vi "TCP Msg Write.vi"(7 "RT":bool, 8 "error in":errorcluster, 9 "timeout ms (10000)":i32=10000, 10 "Packet Info In":T1={"Packet Signature"="", "Sequence Number"=0, "Command"=enum."xml Set LC Input Logic", "Data Message Size"=0, "Data Message Size"="", "Data Message"="", "Error Message Size"=0, "Error Message Size"="", "Error Message"="", "Checksum"=0, "Error Message"={"status"=FALSE, "code"=0, "source"=""}, "Command ID"=""}, 11 "connection ID In":refnum<k5>) -> (0 "error out":errorcluster, 2 "Packet Info In Out":T1={"Packet Signature"="", "Sequence Number"=0, "Command"=enum."Get Info", "Data Message Size"=0, "Data Message Size"="", "Data Message"="", "Error Message Size"=0, "Error Message Size"="", "Error Message"="", "Checksum"=0, "Error Message"={"status"=FALSE, "code"=0, "source"=""}, "Command ID"=""}, 3 "connection ID out":refnum<k5>)   [LabVIEW 2018]
doc: "Writes a package of data to a remote computer via TCP/IP. The VI appends an ID number to each packet. This ID number is used by the Comm TCP Read VI to parse the packet using the meta data. This technique allows appending variable name and type to each packet for ease of use while minimizing the transmission overhead.\n\nThe data must be passed in as a String. The user is responsible for casting or flattening the desired data into a String before passing it to this VI. \n\n* Use the same method for converting to/from String on both the Read and Write functions. For example, if you use the 'Cast' primitive to convert the data into a String, make sure that the 'Cast' primitive is used on the receiving side to convert the data from String to its original form."
uses:
  Type Defs/TCP Packet Info.ctl
  Type Defs/RT Command.ctl
  Type Defs/TCP Packet Parsing State Machine.ctl
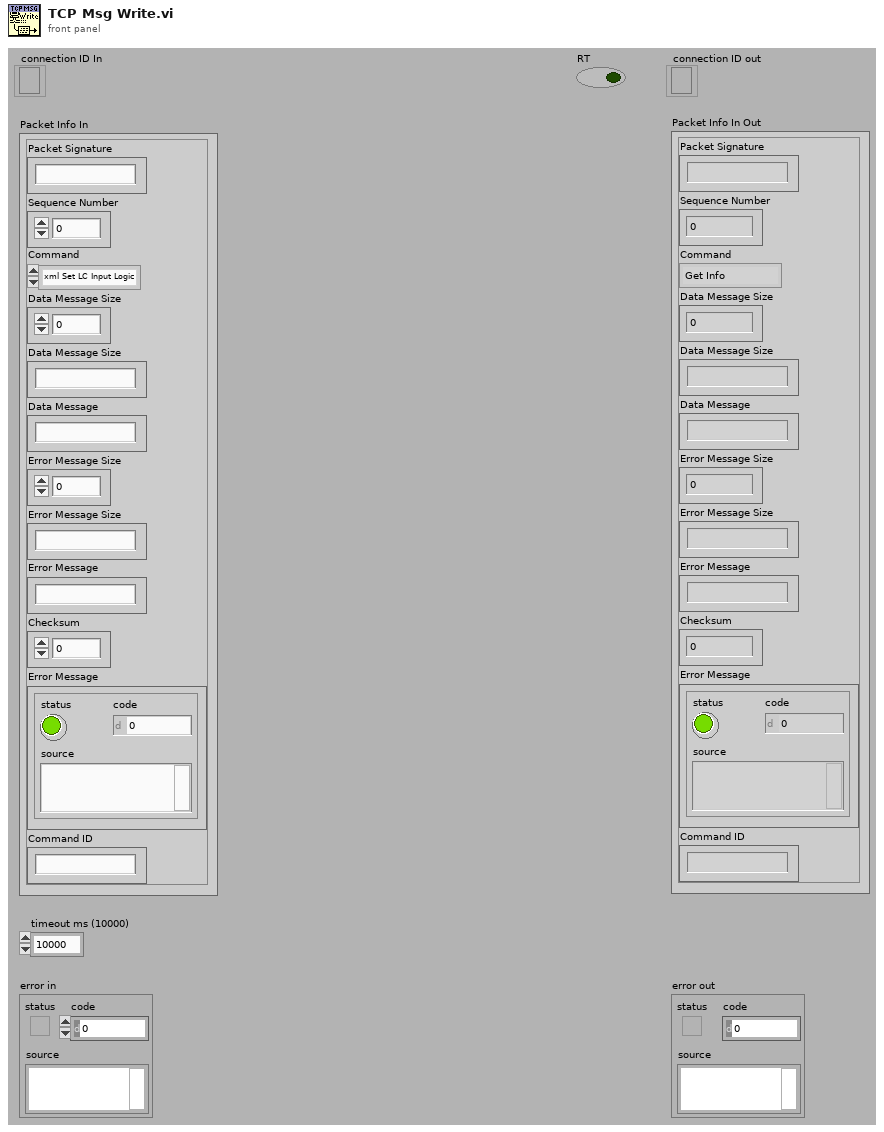
[diagram p1: front panel]
types:
  T1 = typedef "TCP Packet Info.ctl" = cluster{"Packet Signature":string, "Sequence Number":i32, "Command":T2, "Data Message Size":u32, "Data Message Size":string, "Data Message":string, "Error Message Size":u32, "Error Message Size":string, "Error Message":string, "Checksum":u32, "Error Message":errorcluster, "Command ID":string}
  T2 = typedef "RT Command.ctl" = enum16{"xml Start Run", "xml Start Actual Run", "xml Stop Run", "xml Runtime Update", "xml Get Status", "xml Get Table", "xml Set Table", "xml Get Configuration", "xml System Status", "xml Set LC Input Logic", "xml Get Data", "xml Get Info", "Start", "StartActualRun", "Stop", "Runtime Update", "Get Data", "Get Info", "Get Status", "Get Param", "Get Config", "Get Table", "Read ADC", "Set Oscillator", "Update Config", "Update Table", "Set All Pol", "Set Pol and DC", "Set Max Mass", "Toggle RP", "Toggle EL", "Set PIC", "Initialize Turbo", "Send Turbo Comm", "Close Turbo", "P1", "P2", "P3", "Send Serial", "Set LC Out", "Get LC In", "Read VAC", "Test Table", "Toggle Power", "Get Startup", "Set Startup", "Get ADC Table", "Set ADC Table", "Get Brief Status", "Get Detail Status", "Auxiliary Update", "Set CC Logics", "Set CC Input Logics", "Ignore Error", "invalid"}
  T3 = typedef "TCP Packet Parsing State Machine.ctl" = enum16{"Packet Signature", "Sequence Number", "Command ID", "Data Message Size", "Data Message", "Error Message Size", "Error Message", "Checksum", "Invalid Packet Structure"}
  T4 = enum16{"big-endian, network order", "native, host order", "little-endian"}
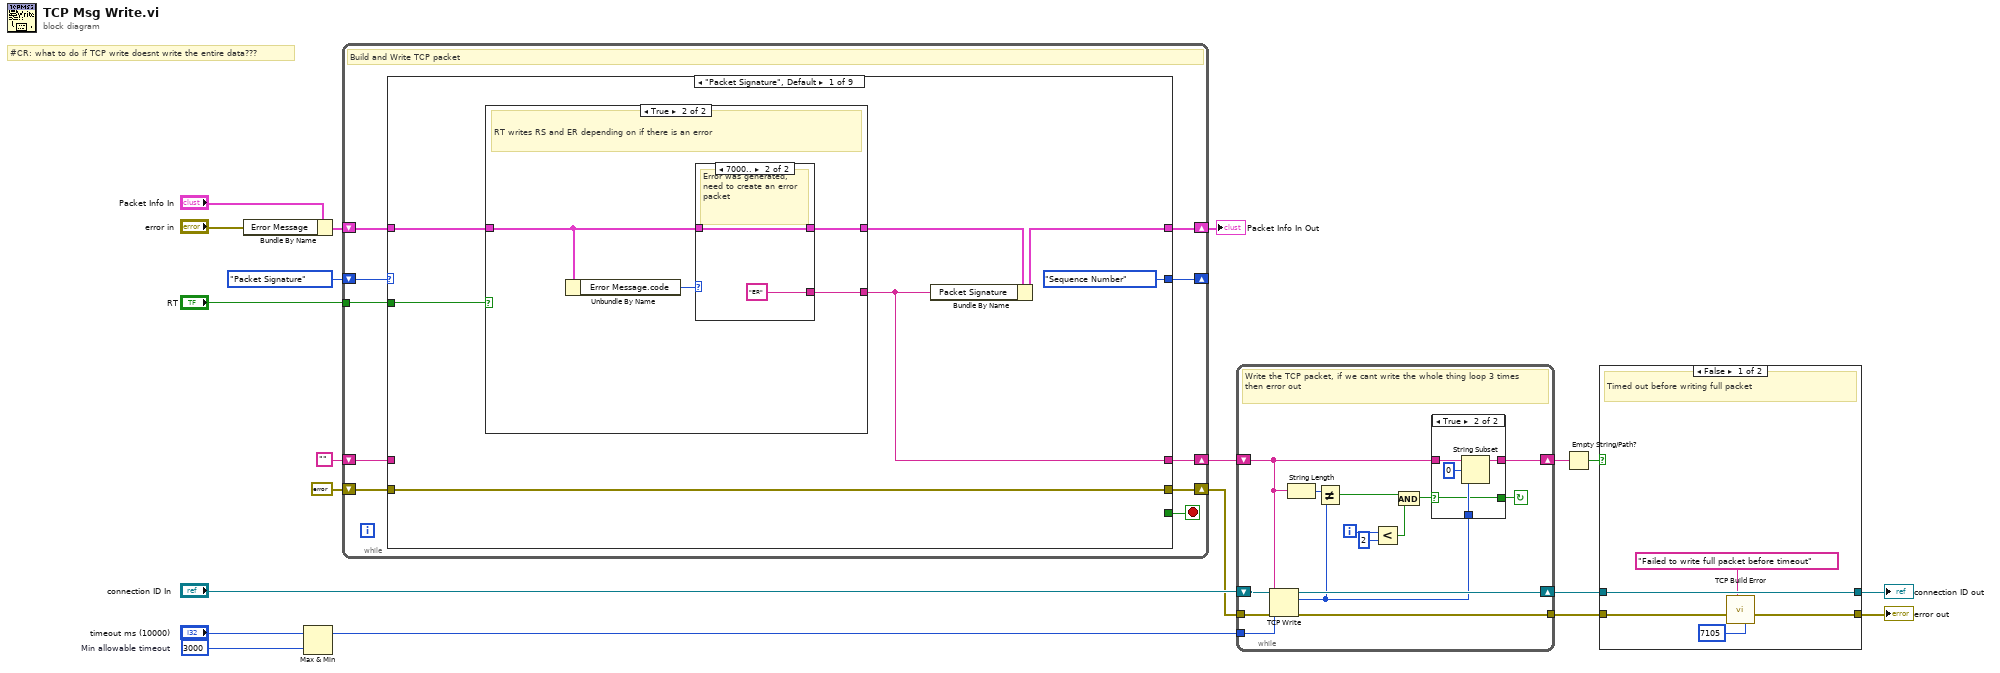
[diagram p0: block diagram]
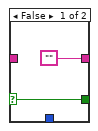
[diagram p3: hidden frame]
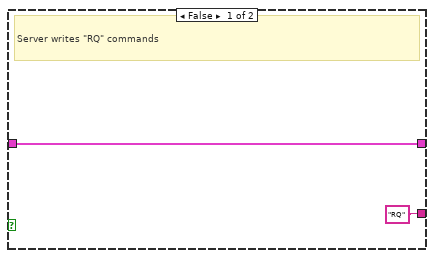
[diagram p4: hidden frame]
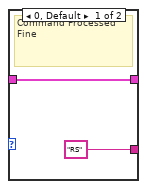
[diagram p5: hidden frame]
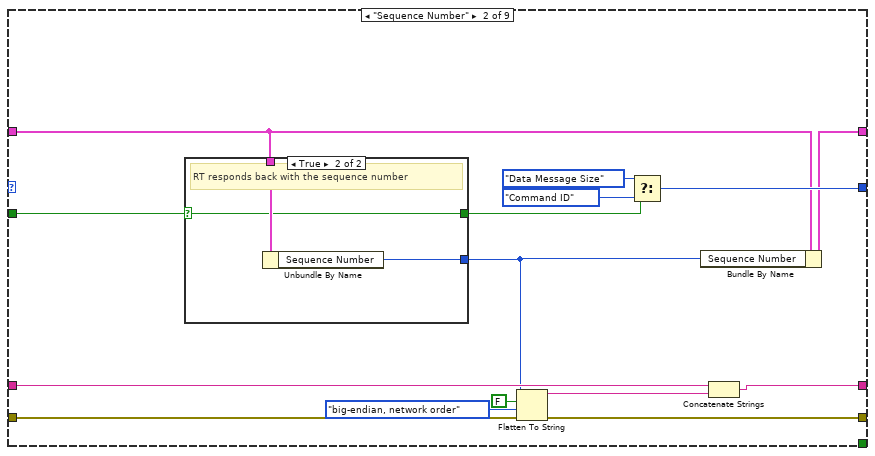
[diagram p6: hidden frame]
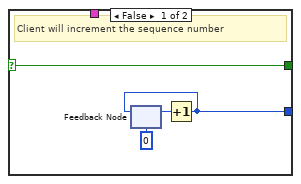
[diagram p7: hidden frame]
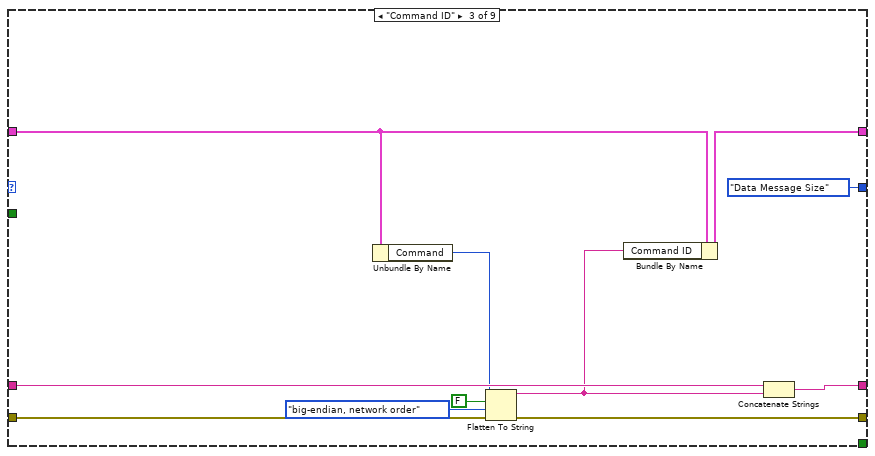
[diagram p8: hidden frame]
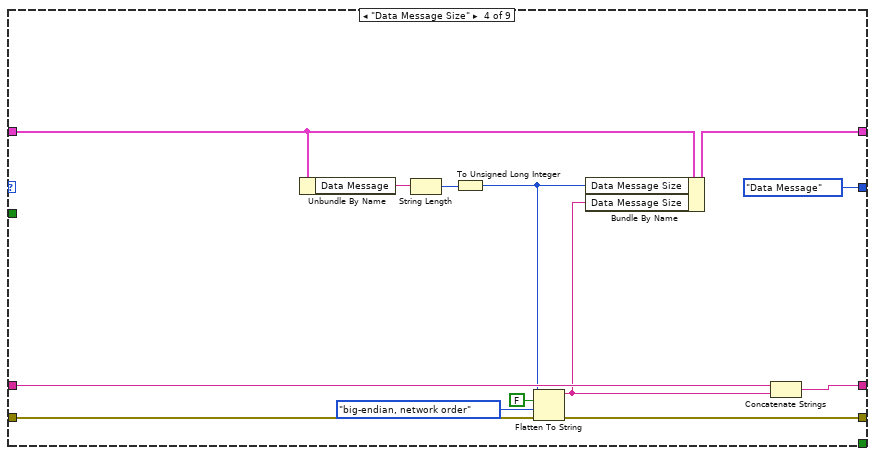
[diagram p9: hidden frame]
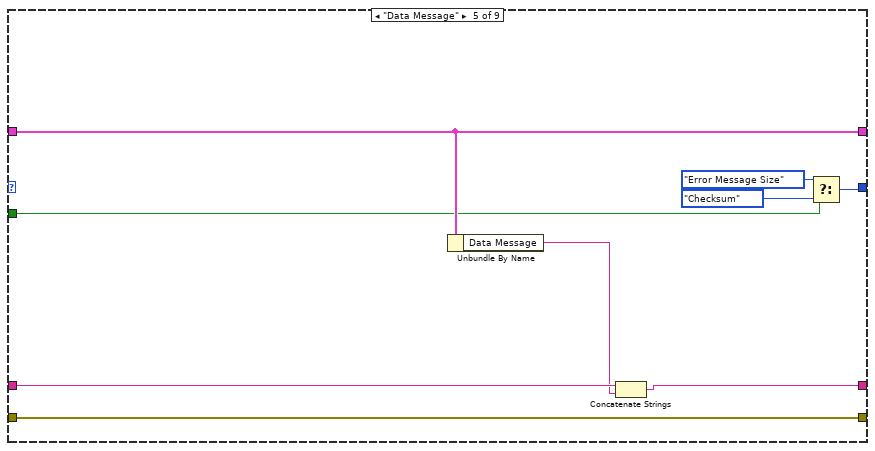
[diagram p10: hidden frame]
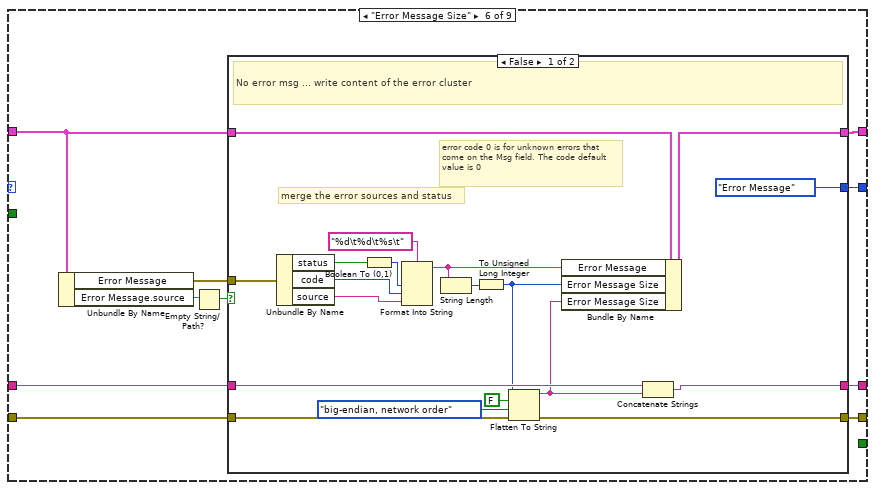
[diagram p11: hidden frame]
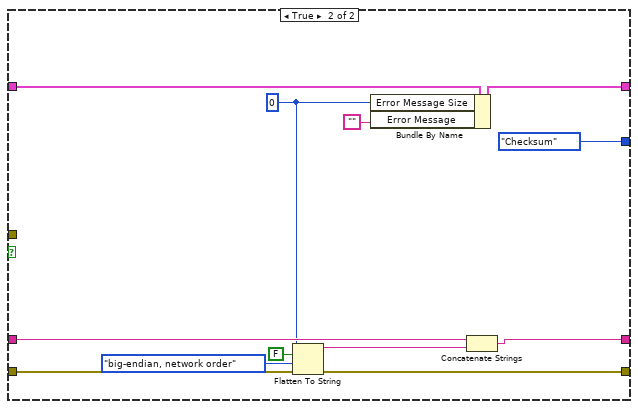
[diagram p12: hidden frame]
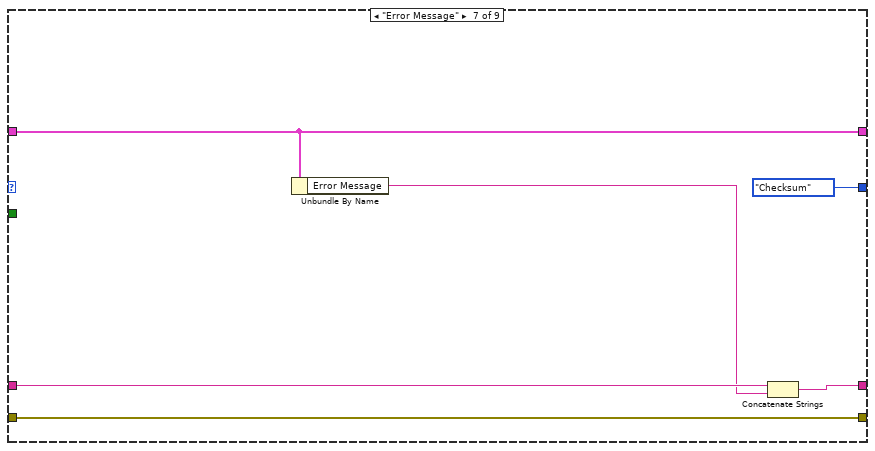
[diagram p13: hidden frame]
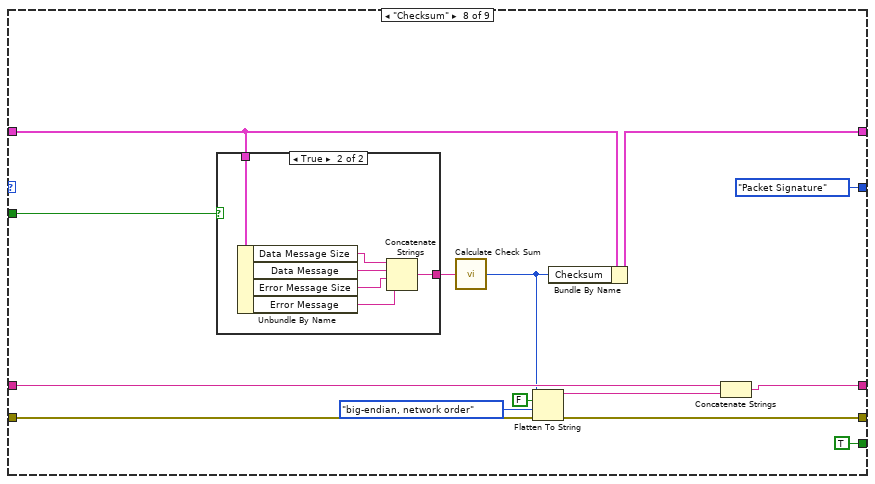
[diagram p14: hidden frame]
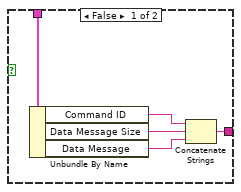
[diagram p15: hidden frame]
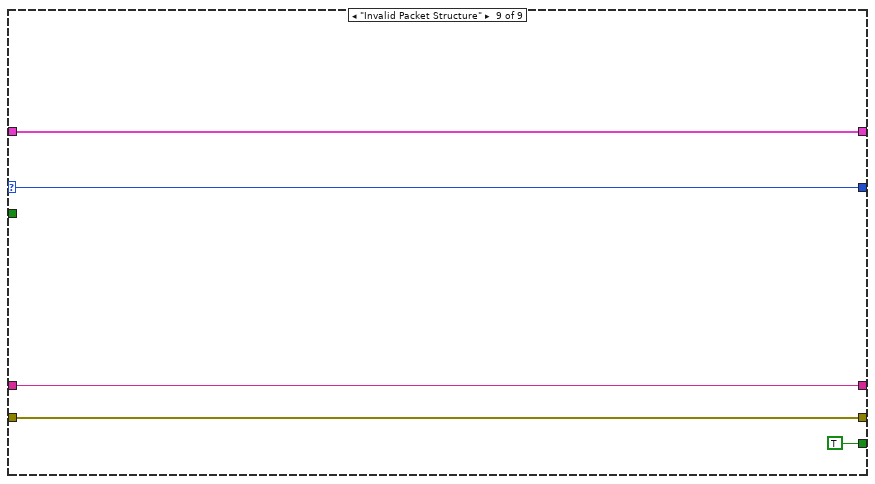
[diagram p16: hidden frame]
diagram:
  w16 = 3000  # Min allowable timeout
  # "#CR: what to do if TCP write doesnt write the entire data???"
  n1 = Bundle By Name(cluster="Packet Info In", "Error Message"="error in") -> (w15:T1)
  n2 = Max & Min(x="timeout ms (10000)", y=w16) -> (max(x,y)=w4:i32)  [unwired: 1 out]
  n3 = while {
    shift-right: [w29] -> w11
    shift-left: w15 -> [w30]
    tunnel: "RT" -> [w28]
    shift-right: [w27] -> _
    shift-left: TCP_Packet_Parsing_State_Machine."Packet Signature" ("Packet Structure") -> [w25]
    shift-right: [w23] -> w3
    shift-left: "" ("Message Packet") -> [w24]
    shift-right: [w21] -> w5
    shift-left: errorcluster {"status"=FALSE, "code"=0, "source"=""} ("error out") -> [w22]
    stop <- w26 stop-if-true
    # "Build and Write TCP packet"
    n4 = case shown="\"Packet Signature\", Default" w25 {
      selector: w25 -> [_ _ _ _ _ _ _ _ w177]
      tunnel: w30 -> [w35 w58 w80 w92 w102 w107 w149 w162 w179]
      tunnel: [w32 w49 w71 w83 w102 w108 w149 w163 w179] -> w29
      tunnel: w28 -> [w37 w59 _ _ w100 _ _ w159 _]
      tunnel: [TCP_Packet_Parsing_State_Machine."Sequence Number" ("Packet Structure") w61 TCP_Packet_Parsing_State_Machine."Data Message Size" ("Packet Structure") TCP_Packet_Parsing_State_Machine."Data Message" ("Packet Structure") w101 w111 TCP_Packet_Parsing_State_Machine."Checksum" ("Packet Structure") TCP_Packet_Parsing_State_Machine."Packet Signature" ("Packet Structure") w177] -> w27
      tunnel: [_ _ _ _ _ _ _ TRUE TRUE] -> w26
      tunnel: w24 -> [_ w56 w78 w88 w97 w106 w147 w157 w176]
      tunnel: [w31 w55 w77 w89 w96 w105 w146 w156 w176] -> w23
      tunnel: w22 -> [w33 w54 w74 w84 w94 w103 w144 w151 w175]
      tunnel: [w33 w51 w73 w85 w94 w104 w144 w153 w175] -> w21
      frame "Packet Signature", Default {
        # "Packet Header"
        n5 = case shown="True" w37 {
          tunnel: w35 -> [w39 w43]
          tunnel: [w39 w42] -> w36
          tunnel: ["RQ" ("data in") w41] -> w31
          frame False {
            # "Server writes \"RQ\" commands"
          }
          frame True {
            # "RT writes RS and ER depending on if there is an error"
            n6 = Unbundle By Name(w43) -> ("Error Message.code"=w40:i32)
            n7 = case shown="7000.." w40 {
              tunnel: w43 -> [w45 w47]
              tunnel: [w45 w47] -> w42
              tunnel: ["RS" ("data in") "ER" ("data in")] -> w41
              frame 0, Default {
                # "Command Processed Fine"
              }
              frame 7000.. {
                # "Error was generated, need to create an error packet"
              }
            }
          }
        }
        n8 = Bundle By Name(cluster=w36, "Packet Signature"=w31) -> (w32:T1)
      }
      frame "Sequence Number" {
        n9 = case shown="True" w59 {
          selector: w59 -> [w63 w67]
          tunnel: w58 -> [_ w69]
          tunnel: [w64 w68] -> w48
          tunnel: [w63 w67] -> w57
          frame False {
            # "Client will increment the sequence number"
            n10 = feedback #1(0 ("Sequence Number")) -> (w65:i32)
            n11 = Increment(x=w65) -> (x+1=w64:i32)
            n12 = feedback-in #1(w64) -> ()
          }
          frame True {
            # "RT responds back with the sequence number"
            n13 = Unbundle By Name(w69) -> ("Sequence Number"=w68:i32)
          }
        }
        n14 = Flatten To String(anything=w48, prepend array or string size? (T)=FALSE, byte order (0:big-endian, network order)=T4."big-endian, network order", error in (no error)=w54) -> (data string=w52:string, error out=w51:errorcluster)  [unwired: 1 out]
        n15 = Select(t=TCP_Packet_Parsing_State_Machine."Data Message Size" ("Packet Structure"), s=w57, f=TCP_Packet_Parsing_State_Machine."Command ID") -> (s? t:f=w61:T3)
        n16 = Bundle By Name(cluster=w58, "Sequence Number"=w48) -> (w49:T1)
        n17 = Concatenate Strings(w56, w52) -> (w55:string)
      }
      frame "Command ID" {
        n18 = Unbundle By Name(w80) -> ("Command"=w72:T2)
        n19 = Flatten To String(anything=w72, prepend array or string size? (T)=FALSE, byte order (0:big-endian, network order)=T4."big-endian, network order", error in (no error)=w74) -> (data string=w70:string, error out=w73:errorcluster)  [unwired: 1 out]
        n20 = Bundle By Name(cluster=w80, "Command ID"=w70) -> (w71:T1)
        n21 = Concatenate Strings(w78, w70) -> (w77:string)
      }
      frame "Data Message Size" {
        n22 = Unbundle By Name(w92) -> ("Data Message"=w91:string)
        n23 = String Length(string=w91) -> (length=w90:i32)
        n24 = To Unsigned Long Integer(number=w90) -> (unsigned 32bit integer=w82:u32)
        n25 = Flatten To String(anything=w82, prepend array or string size? (T)=FALSE ("data includes array or string size? (T)"), byte order (0:big-endian, network order)=T4."big-endian, network order", error in (no error)=w84) -> (data string=w81:string, error out=w85:errorcluster)  [unwired: 1 out]
        n26 = Bundle By Name(cluster=w92, "Data Message Size"=w82, "Data Message Size"=w81) -> (w83:T1)
        n27 = Concatenate Strings(w88, w81) -> (w89:string)
      }
      frame "Data Message" {
        n28 = Unbundle By Name(w102) -> ("Data Message"=w95:string)
        n29 = Concatenate Strings(w97, w95) -> (w96:string)
        n30 = Select(t=TCP_Packet_Parsing_State_Machine."Error Message Size" ("f"), s=w100, f=TCP_Packet_Parsing_State_Machine."Checksum" ("Packet Structure")) -> (s? t:f=w101:T3)
      }
      frame "Error Message Size" {
        n31 = Unbundle By Name(w107) -> ("Error Message"=w110:errorcluster, "Error Message.source"=w109:string)
        n32 = Empty String/Path?(string/path=w109) -> (empty?=w112:bool)
        n33 = case shown="False" w112 {
          tunnel: [TCP_Packet_Parsing_State_Machine."Error Message" ("Packet Structure") TCP_Packet_Parsing_State_Machine."Checksum" ("Packet Structure")] -> w111
          tunnel: w110 -> [w130 _]
          tunnel: [w124 w135] -> w108
          tunnel: w107 -> [w125 w142]
          tunnel: w106 -> [w120 w137]
          tunnel: [w119 w136] -> w105
          tunnel: [w117 w138] -> w104
          tunnel: w103 -> [w116 w139]
          frame False {
            # "error code 0 is for unknown errors that \ncome on the Msg field. The code default \nvalue is 0"
            # "merge the error sources and status"
            # "No error msg ... write content of the error cluster"
            n34 = Unbundle By Name(w130) -> ("status"=w121:bool, "code"=w127:i32, "source"=w126:string)
            n35 = Boolean To (0,1)(Boolean=w121) -> (0, 1=w128:i16)
            n36 = Format Into String(format string="%d\t%d\t%s\t", w128, w127, w126) -> (resulting string=w123:string)  [unwired: 2 in, 1 out]
            n37 = String Length(string=w123) -> (length=w122:i32)
            n38 = To Unsigned Long Integer(number=w122) -> (unsigned 32bit integer=w114:u32)
            n39 = Flatten To String(anything=w114, prepend array or string size? (T)=FALSE ("data includes array or string size? (T)"), byte order (0:big-endian, network order)=T4."big-endian, network order", error in (no error)=w116) -> (data string=w113:string, error out=w117:errorcluster)  [unwired: 1 out]
            n40 = Bundle By Name(cluster=w125, "Error Message"=w123, "Error Message Size"=w114, "Error Message Size"=w113) -> (w124:T1)
            n41 = Concatenate Strings(w120, w113) -> (w119:string)
          }
          frame True {
            w134 = u32 0 ("unsigned 32bit integer")
            n42 = Flatten To String(anything=w134, prepend array or string size? (T)=FALSE ("data includes array or string size? (T)"), byte order (0:big-endian, network order)=T4."big-endian, network order", error in (no error)=w139) -> (data string=w133:string, error out=w138:errorcluster)  [unwired: 1 out]
            n43 = Bundle By Name(cluster=w142, "Error Message Size"=w134, "Error Message"="") -> (w135:T1)
            n44 = Concatenate Strings(w137, w133) -> (w136:string)
          }
        }
      }
      frame "Error Message" {
        n45 = Unbundle By Name(w149) -> ("Error Message"=w145:string)
        n46 = Concatenate Strings(w147, w145) -> (w146:string)
      }
      frame "Checksum" {
        n47 = case shown="True" w159 {
          tunnel: w162 -> [w168 w174]
          tunnel: [w164 w173] -> w161
          frame False {
            n48 = Unbundle By Name(w168) -> ("Command ID"=w167:string, "Data Message Size"=w166:string, "Data Message"=w165:string)
            n49 = Concatenate Strings(w167, w166, w165) -> (w164:string)
          }
          frame True {
            n50 = Unbundle By Name(w174) -> ("Data Message Size"=w172:string, "Data Message"=w171:string, "Error Message Size"=w170:string, "Error Message"=w169:string)
            n51 = Concatenate Strings(w172, w171, w170, w169) -> (w173:string)
          }
        }
        n52 = call "Calculate Check Sum.vi"("Stream"=w161) -> ("Checksum"=w150:u32)
        n53 = Flatten To String(anything=w150, prepend array or string size? (T)=FALSE ("data includes array or string size? (T)"), byte order (0:big-endian, network order)=T4."big-endian, network order", error in (no error)=w151) -> (data string=w152:string, error out=w153:errorcluster)  [unwired: 1 out]
        n54 = Bundle By Name(cluster=w162, "Checksum"=w150) -> (w163:T1)
        n55 = Concatenate Strings(w157, w152) -> (w156:string)
      }
      frame "Invalid Packet Structure" {
      }
    }
  }
  "Packet Info In Out" <- w11
  n56 = while {
    tunnel: w4 -> [w191]
    shift-right: [w194] -> w10
    shift-left: "connection ID In" -> [w192]
    shift-right: [w189] -> w2
    shift-left: w3 -> [w187]
    tunnel: w5 -> [w190]
    tunnel: [w193] -> w9
    i -> [w184]
    stop <- w188 continue-if-true
    # "Write the TCP packet, if we cant write the whole thing loop 3 times then error out"
    n57 = TCP Write(connection ID=w192, data in=w187, error in (no error)=w190, 9:w191) -> (connection ID out=w194:refnum<k5>, bytes written=w185:i32, error out=w193:errorcluster)
    n58 = String Length(string=w187) -> (length=w186:i32)
    n59 = Not Equal?(x=w186, y=w185) -> (x != y?=w182:bool)
    n60 = Less?(x=w184, y=2) -> (x < y?=w180:bool)
    n61 = And(x=w182, y=w180) -> (x .and. y?=w181:bool)
    n62 = case shown="True" w181 {
      selector: w181 -> [w196 w197]
      tunnel: ["" w198] -> w189
      tunnel: w187 -> [_ w199]
      tunnel: [w196 w197] -> w188
      tunnel: w185 -> [_ w200]
      frame False {
      }
      frame True {
        n63 = String Subset(string=w199, offset (0)=0, length (rest)=w200) -> (substring=w198:string)
      }
    }
  }
  n64 = Empty String/Path?(string/path=w2) -> (empty?=w1:bool)
  n65 = case shown="False" w1 {
    tunnel: w9 -> [w205 w207]
    tunnel: [w206 w208] -> w8
    tunnel: w10 -> [w206 w208]
    tunnel: [w204 w207] -> w7
    frame False {
      # "Timed out before writing full packet"
      n66 = call "TCP Build Error.vi"("code"=7105, "Error"="Failed to write full packet before timeout", "error in (no error)"=w205) -> ("error out"=w204:errorcluster)  [unwired: 8 in]
    }
    frame True {
      # "everything was written"
    }
  }
  "error out" <- w7
  "connection ID out" <- w8
